vi "Initialize.vi"(8 "error in (no error)":errorcluster, 11 "Component UI in":refnum<class "DSF Buffer Converter User Interfaces.lvclass">) -> (0 "error out":errorcluster, 3 "Component UI out":refnum<class "DSF Buffer Converter User Interfaces.lvclass">)   [LabVIEW 2017, in "DSF Core.lvlib" / "DSF Buffer Converter User Interfaces.lvclass"]
uses:
  DSF Buffer Converter User Interfaces.lvclass
  C:/Git/DSF/Core/Classes/Component User Interface/Component User Interfaces.lvclass
  Transfer/DSF Buffer Converter Transfers UI.lvclass
  C:/Git/DSF/Core/Classes/User Interface/User Interface.lvclass
  Classes/Component User Interface/Component User Interfaces.lvclass
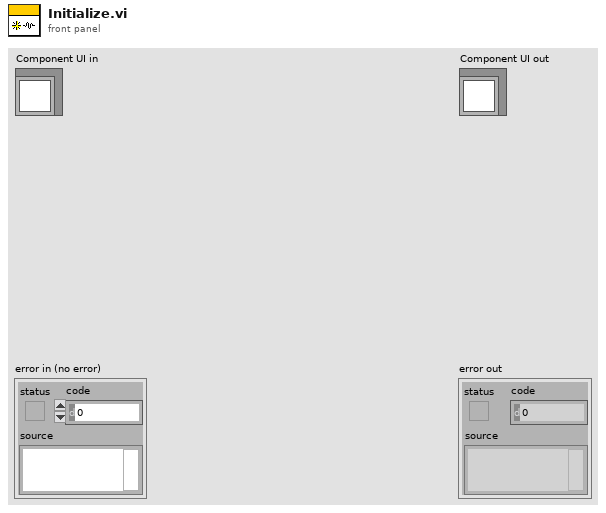
[diagram p1: front panel]
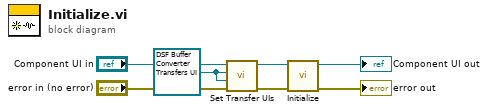
[diagram p0: block diagram]
diagram:
  w5 = refnum<class "DSF Buffer Converter Transfers UI.lvclass"> refnum ("DSF Core.lvlib:DSF Buffer Converter Transfers UI.lvclass")
  n1 = call "Set Transfer UIs.vi"("error in (no error)"="error in (no error)", "Tx Transfer UI"=w5, "Rx Transfer UI"=w5, "Component UI in"="Component UI in") -> ("error out"=w3:errorcluster, "Component UI out"=w4:refnum<class "DSF Buffer Converter User Interfaces.lvclass">)  [unwired: 6 in]
  n2 = call-parent "Initialize.vi"("error in (no error)"=w3, "Component UI in"=w4) -> ("error out"=→"error out":errorcluster, "Component UI out"=→"Component UI out":refnum<class "DSF Buffer Converter User Interfaces.lvclass">)  [unwired: 8 in]
